vi "cDAQ DDS Process.vi"(8 "error in":errorcluster, 11 "session in":variant) -> (0 "error out":errorcluster)   [LabVIEW 2020]
uses:
  cDAQ DDS Session.ctl
  cDAQ DDS Setup.ctl
  cDAQ DDS Timebase Mode.ctl
  <vilib>/DAQmx/write.llb/DAQmx Write (Analog 2D DBL NChan NSamp).vi
  <vilib>/DAQmx/miscellaneous.llb/DAQmx Fill In Error Info.vi
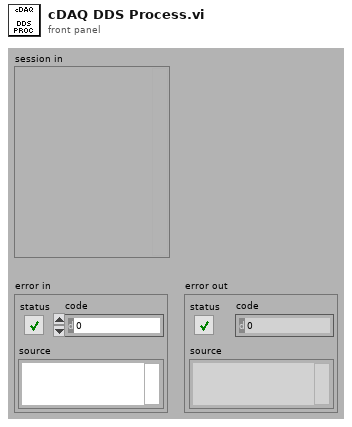
[diagram p1: front panel]
types:
  T1 = typedef "cDAQ DDS Setup.ctl" = cluster{"A [V]":dbl[], "ph [rad]":dbl[], "f [Hz]":dbl[], "stop":bool, "ofs [V]":dbl[]}
  T2 = typedef "cDAQ DDS Session.ctl" = cluster{"device":tag, "channels":i32[], "mclk source":tag, "mclk [Hz]":dbl, "fs [Hz]":dbl, "block [s]":dbl, "buf [s]":dbl, "task":refnum<k21>, "cmd queue":refnum<queue>, "proc ref":refnum<vi>, "smpl clock out":tag, "export smpl clock":bool, "DC ofs [V]":dbl[], "timebase source":tag, "timebase mode":T3}
  T3 = typedef "cDAQ DDS Timebase Mode.ctl" = enum16{"Local", "Take from ADC (e.g. NI 9238)", "Other source"}
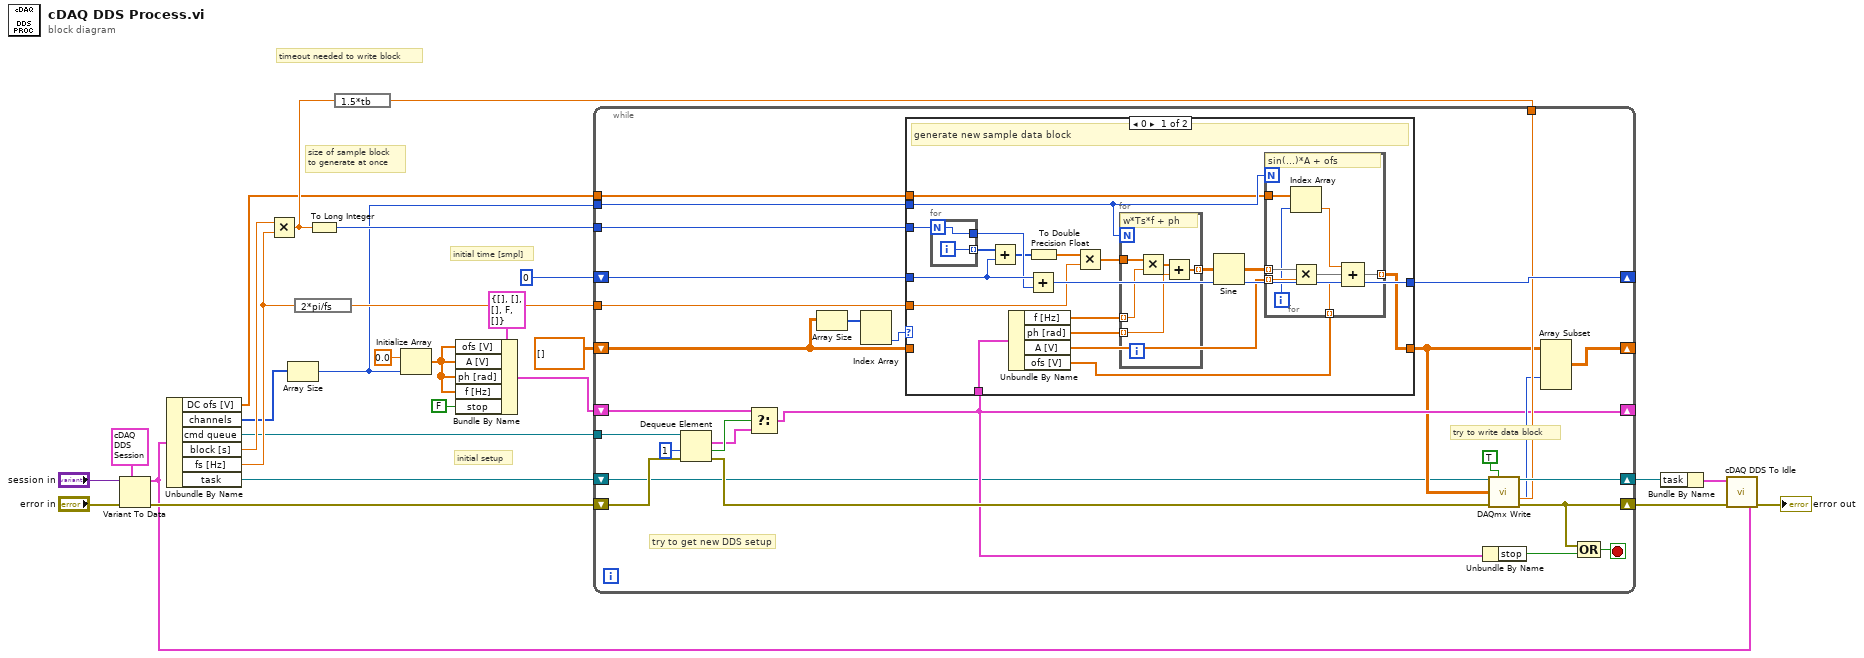
[diagram p0: block diagram]
diagram:
  # "initial setup"
  # "initial time [smpl]"
  # "timeout needed to write block"
  # "size of sample block\nto generate at once"
  n1 = Variant To Data(error in="error in", type=T2 {"device"="", "channels"=[], "mclk source"="", "mclk [Hz]"=0.0, "fs [Hz]"=0.0, "block [s]"=0.0, "buf [s]"=0.0, "task"="", "cmd queue"=refnum, "proc ref"=refnum, "smpl clock out"="", "export smpl clock"=FALSE, "DC ofs [V]"=[], "timebase source"="", "timebase mode"=enum."Local"} ("cDAQ dds"), Variant="session in") -> (data=w7:T2, error out=w24:errorcluster)
  n2 = Unbundle By Name(w7) -> ("DC ofs [V]"=w1:dbl[], "channels"=w14:i32[], "cmd queue"=w15:refnum<queue>, "block [s]"=w21:dbl, "fs [Hz]"=w20:dbl, "task"=w23:refnum<k21>)
  n3 = Multiply(x=w21, y=w20) -> (x*y=w18:dbl)
  n4 = Array Size(array=w14) -> (size(s)=w3:i32)
  n5 = expression code="2*pi/fs"(w20) -> (w22:dbl)
  n6 = To Long Integer(number=w18) -> (32bit integer=w19:i32)
  n7 = expression code="1.5*tb"(w18) -> (w17:dbl)
  n8 = Initialize Array(0.0 ("element"), w3) -> (w2:dbl[])
  n9 = Bundle By Name(cluster=T1 {"A [V]"=[], "ph [rad]"=[], "f [Hz]"=[], "stop"=FALSE, "ofs [V]"=[]} ("cDAQ dds setup"), "ofs [V]"=w2, "A [V]"=w2, "ph [rad]"=w2, "f [Hz]"=w2, "stop"=FALSE) -> (w12:T1)
  n10 = while {
    shift-right: [w47] -> w8
    shift-left: w24 -> [w43]
    shift-right: [w53] -> w6
    shift-left: w23 -> [w29]
    shift-right: [w51] -> _
    shift-left: i64 0 -> [w52]
    shift-right: [w50] -> _
    shift-left: dbl[][] [] -> [w49]
    tunnel: w19 -> [w46]
    tunnel: w17 -> [w45]
    tunnel: w22 -> [w44]
    tunnel: w15 -> [w42]
    shift-right: [w34] -> _
    shift-left: w12 -> [w38]
    tunnel: w3 -> [w32]
    tunnel: w1 -> [w28]
    stop <- w48 stop-if-true
    # "try to write data block"
    # "try to get new DDS setup"
    n11 = Dequeue Element(queue=w42, timeout in ms (-1)=1, error in (no error)=w43) -> (element=w39:T1, timed out?=w40:bool, error out=w37:errorcluster)  [unwired: 1 out]
    n12 = Select(t=w38, s=w40, f=w39) -> (s? t:f=w34:T1)
    n13 = Array Size(array=w49) -> (size(s)=w35:i32[])
    n14 = Index Array(array=w35) -> (element #2=w30:i32)  [unwired: 2 in, 1 out]
    n15 = case shown="0" w30 {
      tunnel: w52 -> [w71 w90]
      tunnel: [w58 w89] -> w31
      tunnel: [w69 w90] -> w51
      tunnel: w49 -> [_ w89]
      tunnel: w46 -> [w73 _]
      tunnel: w44 -> [w66 _]
      tunnel: w34 -> [w65 _]
      tunnel: w32 -> [w57 _]
      tunnel: w28 -> [w55 _]
      frame 0 {
        # "generate new sample data block"
        n16 = for {
          N: w73 -> [w87]
          tunnel: [w88] -> w72 mode=indexing
          tunnel: [w87] -> w70
          i -> [w88]
        }
        n17 = Add(x=w72, y=w71) -> (x+y=w68:i64[])
        n18 = Unbundle By Name(w65) -> ("f [Hz]"=w63:dbl[], "ph [rad]"=w62:dbl[], "A [V]"=w59:dbl[], "ofs [V]"=w56:dbl[])
        n19 = Add(x=w71, y=w70) -> (x+y=w69:i64)
        n20 = To Double Precision Float(number=w68) -> (double precision float=w67:dbl[])
        n21 = Multiply(x=w67, y=w66) -> (x*y=w64:dbl[])
        n22 = for {
          N: w57 -> [_]
          tunnel: w64 -> [w86]
          tunnel: w63 -> [w85] mode=indexing
          tunnel: w62 -> [w83] mode=indexing
          tunnel: [w82] -> w61 mode=indexing
          # "w*Ts*f + ph"
          n23 = Multiply(x=w86, y=w85) -> (x*y=w84:dbl[])
          n24 = Add(x=w84, y=w83) -> (x+y=w82:dbl[])
        }
        n25 = Sine(x=w61) -> (sin(x)=w60:dbl[][])
        n26 = for {
          N: w57 -> [_]
          tunnel: w60 -> [w81] mode=indexing
          tunnel: w59 -> [w80] mode=indexing
          tunnel: [w79] -> w58 mode=indexing
          tunnel: w56 -> [w77] mode=indexing
          tunnel: w55 -> [w75]
          i -> [w74]
          # "sin(...)*A + ofs"
          n27 = Index Array(array=w75, index=w74) -> (element=w76:dbl)
          n28 = Multiply(x=w81, y=w80) -> (x*y=w78:dbl[])
          n29 = Compound Arithmetic op=ADD(w76, w78, w77) -> (w79:dbl[])
        }
      }
      frame Default {
      }
    }
    n30 = Unbundle By Name(w34) -> ("stop"=w33:bool)
    n31 = call-poly <vilib>:"DAQmx Write.vi"("task/channels in"=w29, "auto start"=TRUE, "data"=w31, "timeout"=w45, "error in"=w37) -> ("task out"=w53:refnum<k21>, "number of samples written per channel"=w36:u32, "error out"=w47:errorcluster)  [unwired: 8 in]
    n32 = Array Subset(array=w31, index (col)=w36) -> (w50:dbl[][])  [unwired: 3 in]
    n33 = Compound Arithmetic op=OR(w47, w33) -> (w48:bool)
  }
  n34 = Bundle By Name(cluster=w7, "task"=w6) -> (w5:T2)
  n35 = call "cDAQ DDS To Idle.vi"("error in"=w8, "cDAQ dds"=w5) -> ("error out"=→"error out":errorcluster)  [unwired: 8 in, 1 out]
